vi "TrajectoryConfig_setVoltageDiffDrive.vi"(8 "SIMPLE_MOTOR_FF":T1 {"Ka" format="%13.4f"; "Kv" format="%13.4f"; "Ks" format="%13.4f"}, 9 "DIFF_DRIVE_KINEMATICS":T2 {"TrackWidth_Meters" format="%20.4f"}, 10 "Max Voltage":dbl format="%20.4f", 11 "inTRAJECTORY_CONFIG":T3 {"End Velocity" format="%20.4f"; "StartVelocity" format="%20.4f"; "Max Acceleration" format="%20.4f"; "MaxVelocity" format="%20.4f"}) -> (3 "outTRAJECTORY_CONFIG":T3 {"End Velocity" format="%20.4f"; "StartVelocity" format="%20.4f"; "Max Acceleration" format="%20.4f"; "MaxVelocity" format="%20.4f"})   [LabVIEW 2019, in "Trajectory_Library.lvlib"]
doc: "Adds and enabled a differential drive voltage constraint to ensure that no wheel velocity or acceleration of a differential drive goes above the attainable values. \n\nParameters:\n - InTrajectoryConfig - The trajectory configuration data structure\n - maxVoltage - The maximum voltage available to the motors while following the path. Should be somewhat less than the nominal battery voltage (12V) to account for \"voltage sag\" due to current draw.\n - DiffDriveKinematics - A kinematics component describing the drive geometry.\n - SimpleMotorFeedforward - A feedforward component describing the behavior of the drive.\n\nReturns:\n - OutTrajectoryConfig - Modified trajectory configuration data structure"
uses:
  Trajectory_Library.lvlib
  TRAJ_CONFIG.ctl
  DIFF_DRIVE_KINEMATICS.ctl
  SIMPLE_MOTOR_FF.ctl
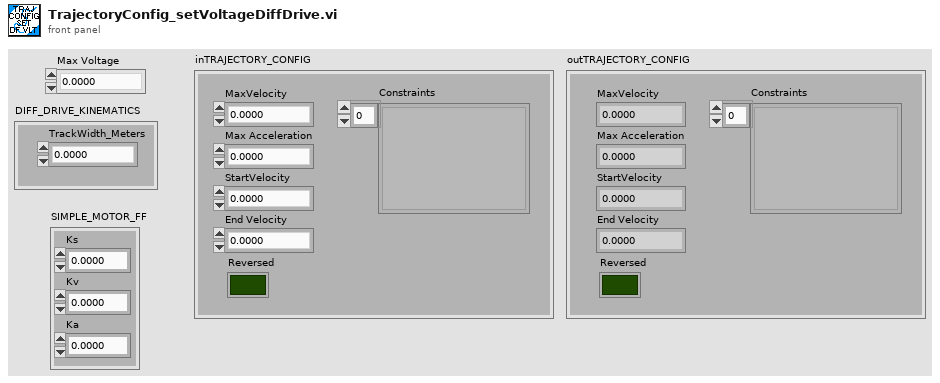
[diagram p1: front panel]
types:
  T1 = typedef "Trajectory_Library.lvlib/SIMPLE_MOTOR_FF.ctl" = cluster{"Ks":dbl, "Kv":dbl, "Ka":dbl}
  T2 = typedef "Trajectory_Library.lvlib/DIFF_DRIVE_KINEMATICS.ctl" = cluster{"TrackWidth_Meters":dbl}
  T3 = typedef "Trajectory_Library.lvlib/TRAJ_CONFIG.ctl" = cluster{"MaxVelocity":dbl, "Max Acceleration":dbl, "StartVelocity":dbl, "End Velocity":dbl, "Reversed":bool, "Constraints":variant[]}
  T4 = typedef "Trajectory_Library.lvlib/TRAJ_CONSTRAINT_DIIF_DRIVE_VOLTAGE.ctl" = cluster{"Max Voltage":dbl, "DIFF_DRIVE_KINEMATICS":T2, "SIMPLE_MOTOR_FF":T1}
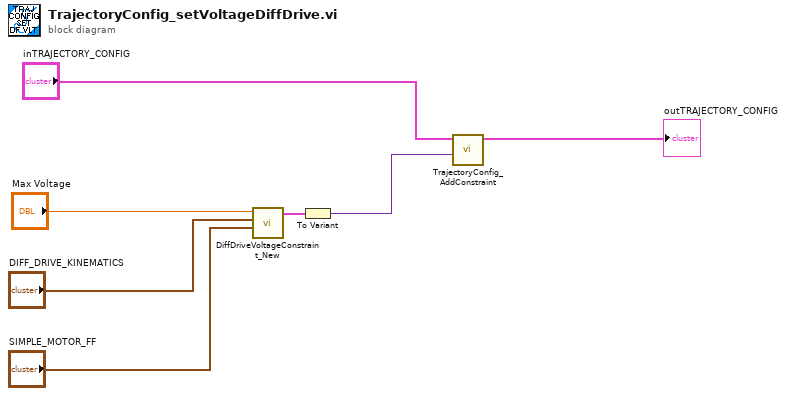
[diagram p0: block diagram]
diagram:
  n1 = call "DiffDriveVoltageConstraint_New.vi"("SIMPLE_MOTOR_FF"="SIMPLE_MOTOR_FF", "DIFF_DRIVE_KINEMATICS"="DIFF_DRIVE_KINEMATICS", "Max Voltage"="Max Voltage") -> ("DIFF_DRIVE_VOLTAGE_CONSTRAINT"=w2:T4)  [unwired: 8 in]
  n2 = To Variant(anything=w2) -> (Variant=w1:variant)
  n3 = call "TrajectoryConfig_AddConstraint.vi"("Constraint"=w1, "inTRAJECTORY_CONFIG"="inTRAJECTORY_CONFIG") -> ("outTRAJECTORY_CONFIG"=→"outTRAJECTORY_CONFIG":T3)  [unwired: 9 in]
